vi "HelperTemplate.vi"(9 "Module":refnum<class>, 10 "Message Queue":refnum<class "ModuleQueue.lvclass">, 11 "ModuleRequests":refnum<user-event>) -> ()   [LabVIEW 2024, in "AddHelper.lvlib"]
uses:
  AddHelper.lvlib
  RQMHCore/ModQueue/ModuleQueue.lvclass
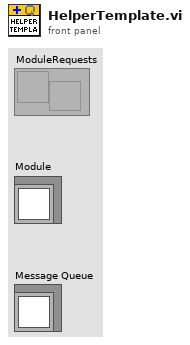
[diagram p1: front panel]
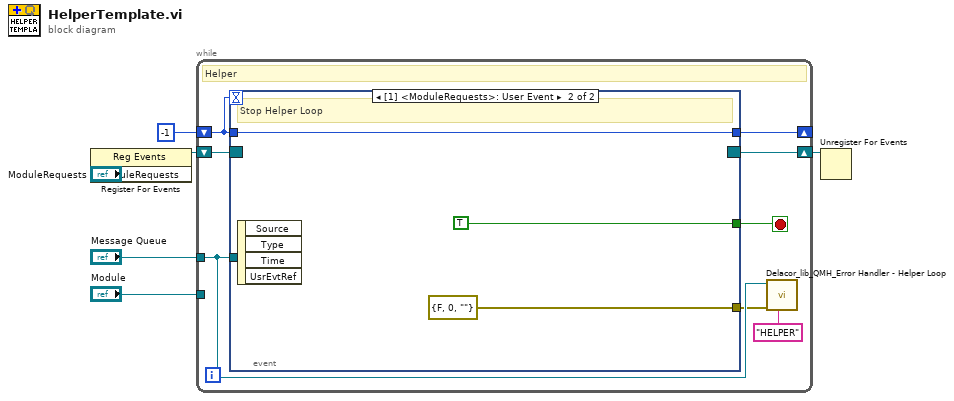
[diagram p0: block diagram]
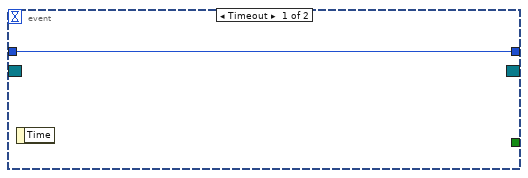
[diagram p2: hidden frame]
diagram:
  n1 = register-events ("DQMH_HELPER_REGFOREVENTS")("ModuleRequests") -> (reference out=w5:refnum<event-registration>)  [unwired: 2 in, 1 out]
  n2 = while "RQMH_HELPER_LOOP" {
    shift-right: [w14] -> _
    shift-left: -1 -> [w13]
    shift-right: [w11] -> w6
    shift-left: w5 -> [w12]
    tunnel: "Message Queue" -> [w9]
    tunnel: "Module" -> [_]
    stop <- w10 stop-if-true
    # "Helper"
    n3 = event "RQMH_HELPER_EVENT_STRUCTURE" shown="[1] <ModuleRequests>: User Event" {
      selector: w12 -> [_ _]
      dyn-events: [_ _] -> w11
      timeout: w13 -> [_ _]
      tunnel: w13 -> [w15 w18]
      tunnel: [w15 w18] -> w14
      tunnel: [_ TRUE] -> w10
      tunnel: [_ errorcluster {"status"=FALSE, "code"=0, "source"=""} ("error constant")] -> w7
      tunnel: w9 -> [_ _]
      event Timeout {
        n4 = event-data() -> ()  [unwired: 1 in, 1 out]
      }
      event User Event {
        # "Stop Helper Loop"
        n5 = event-data() -> ()  [unwired: 1 in, 4 out]
      }
    }
    n6 = call-dynamic "Delacor_lib_QMH_Error Handler - Helper Loop.vi"("HelperName"="HELPER" ("RQMH_HELPER_LOOP_NAME"), "error in"=w7, "Message Queue in"=w9) -> ()  [unwired: 7 in, 2 out]
  }
  n7 = Unregister For Events(event registration refnum=w6) -> ()  [unwired: 1 in, 1 out]
